vi "StateMachine.vi"() -> ()   [LabVIEW 2013, in "GP22_TDC_Arduinoed.lvlib"]
uses:
  GP22_TDC_Arduinoed.lvlib
  typedefs/State.ctl
  typedefs/Data.ctl
  <vilib>/Utility/file.llb/Write To Spreadsheet File (DBL).vi
  Public/Globals.vi
  <vilib>/Analysis/NI_AALBase.lvlib
panel:
  in  "VISA resource name":refnum<visa-resource-name>
  in  "Exit":bool
  in  "Tab Control":T1(tab)
  in  "Start calibration":bool
  in  "Save data":bool
  in  "Number of calibration readings":i32=100
  out "Histogram":dynamicdata(graph)
  out "Standard deviation":dbl format="%^_2g"
  out "Mean":dbl format="%^_4g"
  out "Calibration readings":dbl[](array[numeric])
  in  "Wait time (ms)":u32=10
  out "Progress":u8(slide) scale=0.0..100.0
  in  "Auto calibrate? (false)":bool
  in  "Double resolution? (false)":bool
  out "Freq / Hz":dbl format="%^#_6g"
  out "output / s":dbl format="%^#_6g"
  in  "Single Measurement":bool caption="Measure"
  out "MMProgress":u8(slide) scale=0.0..100.0
  out "output/s":dbl[](array[numeric]) format="%^#_6g"
  out "Raw output":dbl[](array[numeric])
  out "Calibration":dbl[](array[numeric])
  out "Multiple Meas. Histogram":dynamicdata(graph) caption="Histogram"
  in  "Time / ms (30000)":u32=30000
  out "Size":i32
  out "Mean Freq / Hz":dbl format="%^#_6g"
  out "Time frac. S.D.":dbl format="%^#_6e"
  out "Mean Time / s":dbl format="%^.3e"
  in  "Time between calibrations (ms)":u32=1000
  in  "Multiple Measurements":bool caption="Measure"
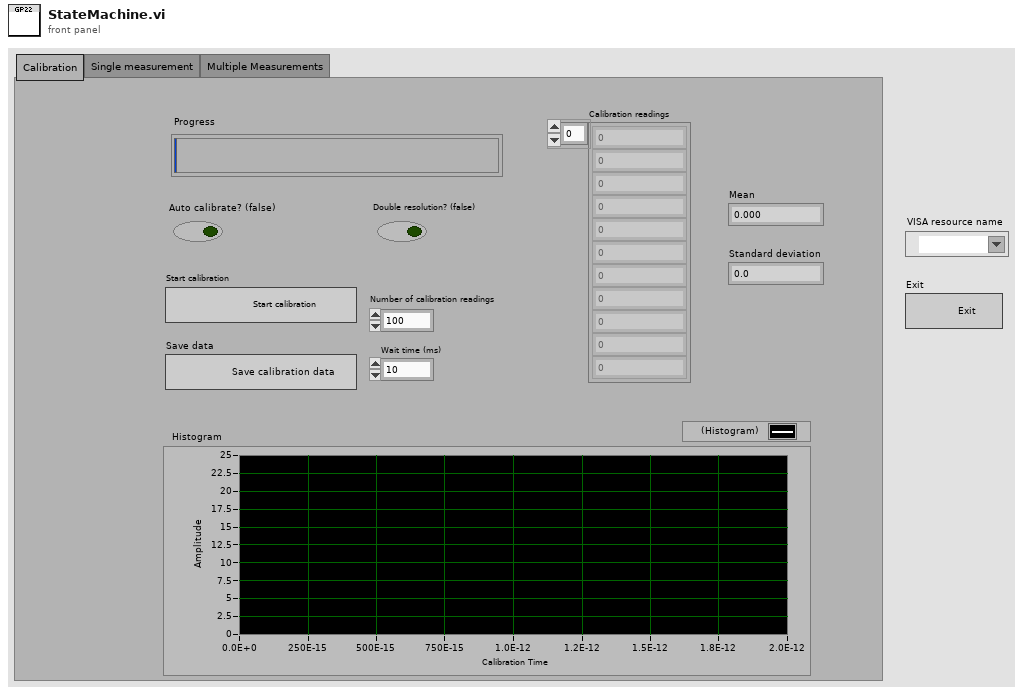
[diagram p1: front panel]
types:
  T1 = enum32{"Calibration", "Single measurement", "Multiple Measurements"}
  T2 = typedef "GP22_TDC_Arduinoed.lvlib/Data.ctl" = cluster{"VISA resource name":refnum<visa-resource-name>}
  T3 = typedef "GP22_TDC_Arduinoed.lvlib/State.ctl" = enum16{"Initialize", "Wait for Event", "Multiple Measurements", "Take calibration data", "Save calibration data", "Single measurement", "Exit"}
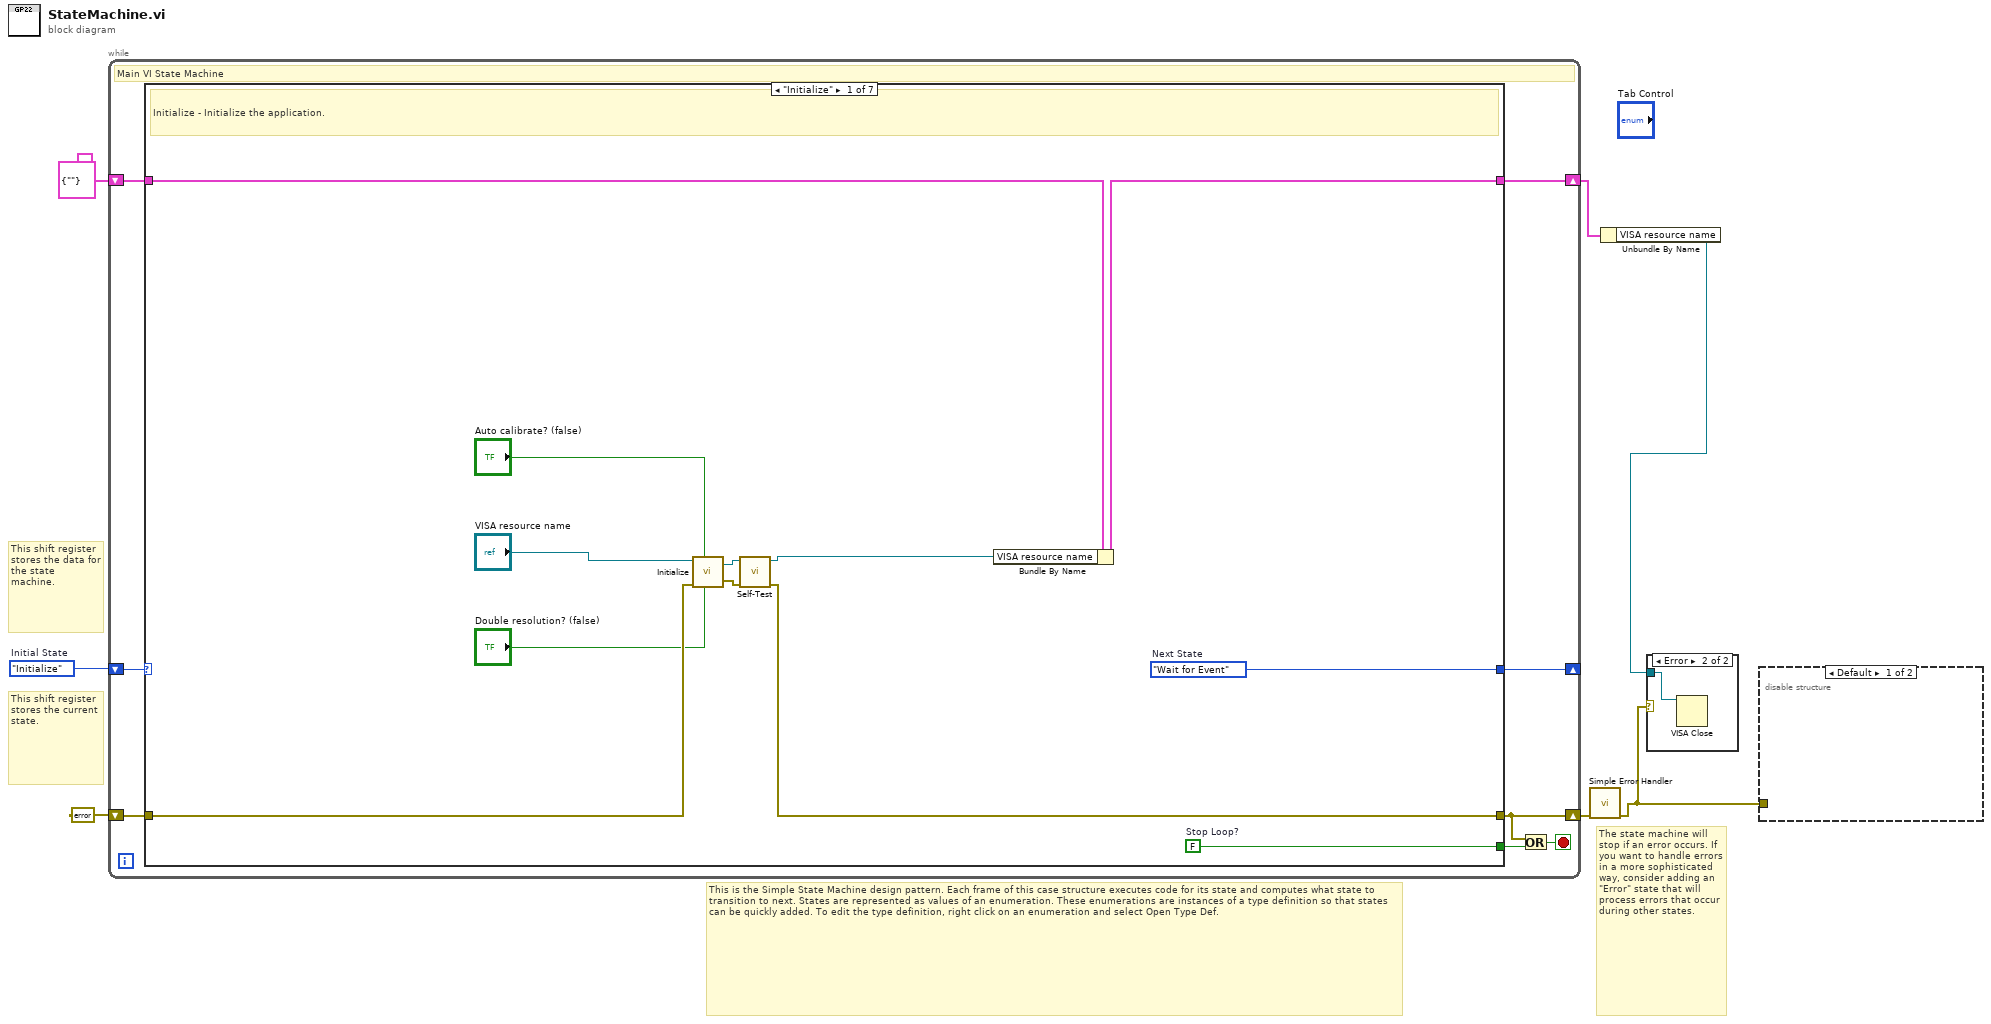
[diagram p0: block diagram]
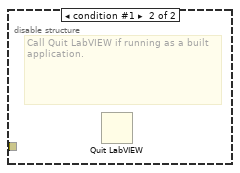
[diagram p3: hidden frame]
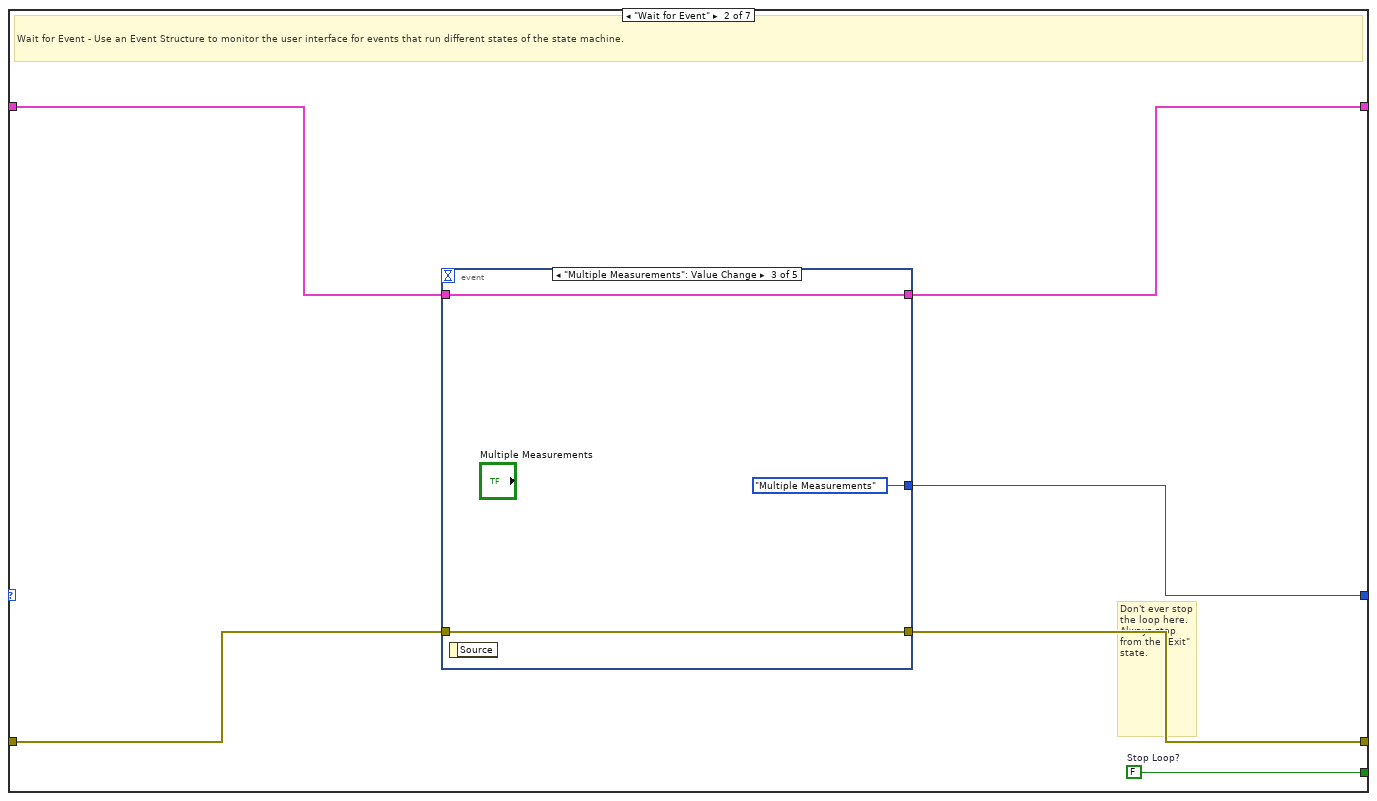
[diagram p4: hidden frame]
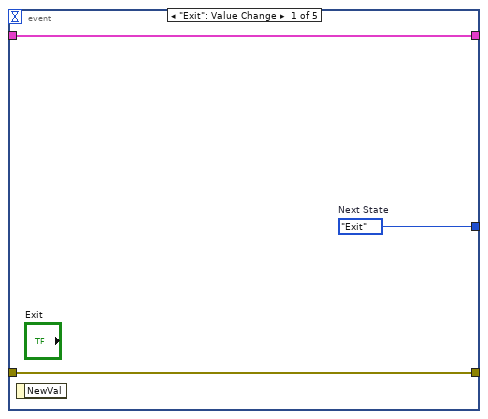
[diagram p5: hidden frame]
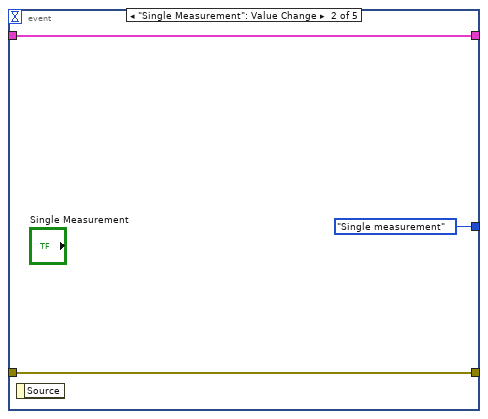
[diagram p6: hidden frame]
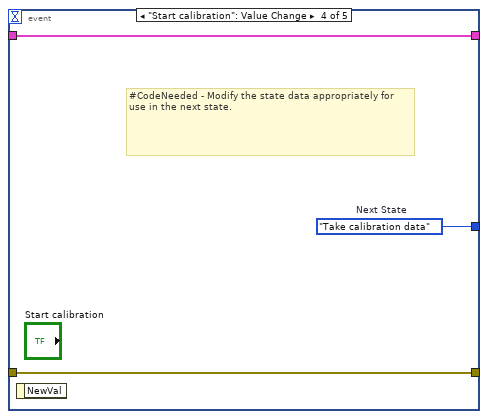
[diagram p7: hidden frame]
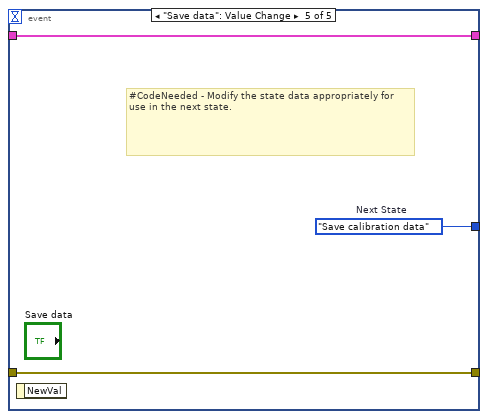
[diagram p8: hidden frame]
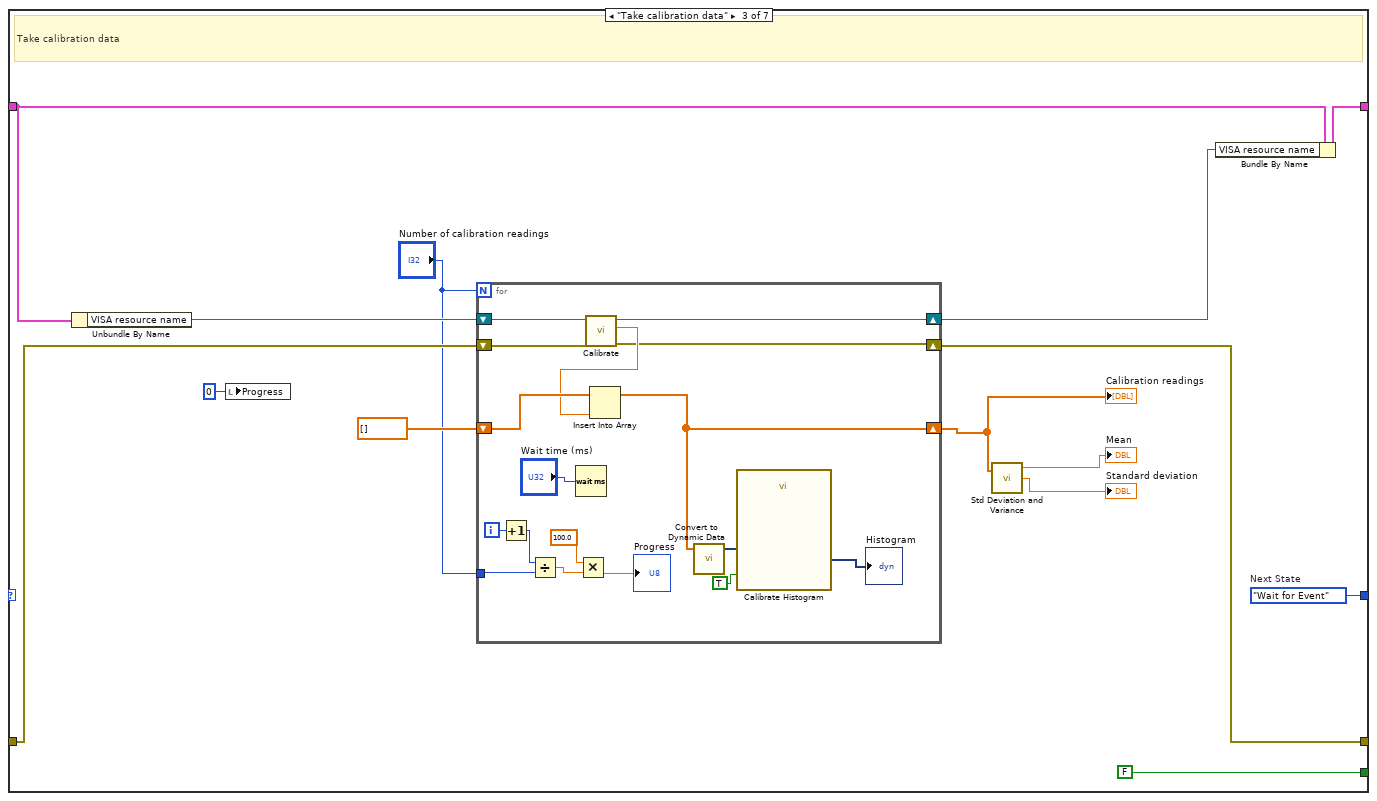
[diagram p9: hidden frame]
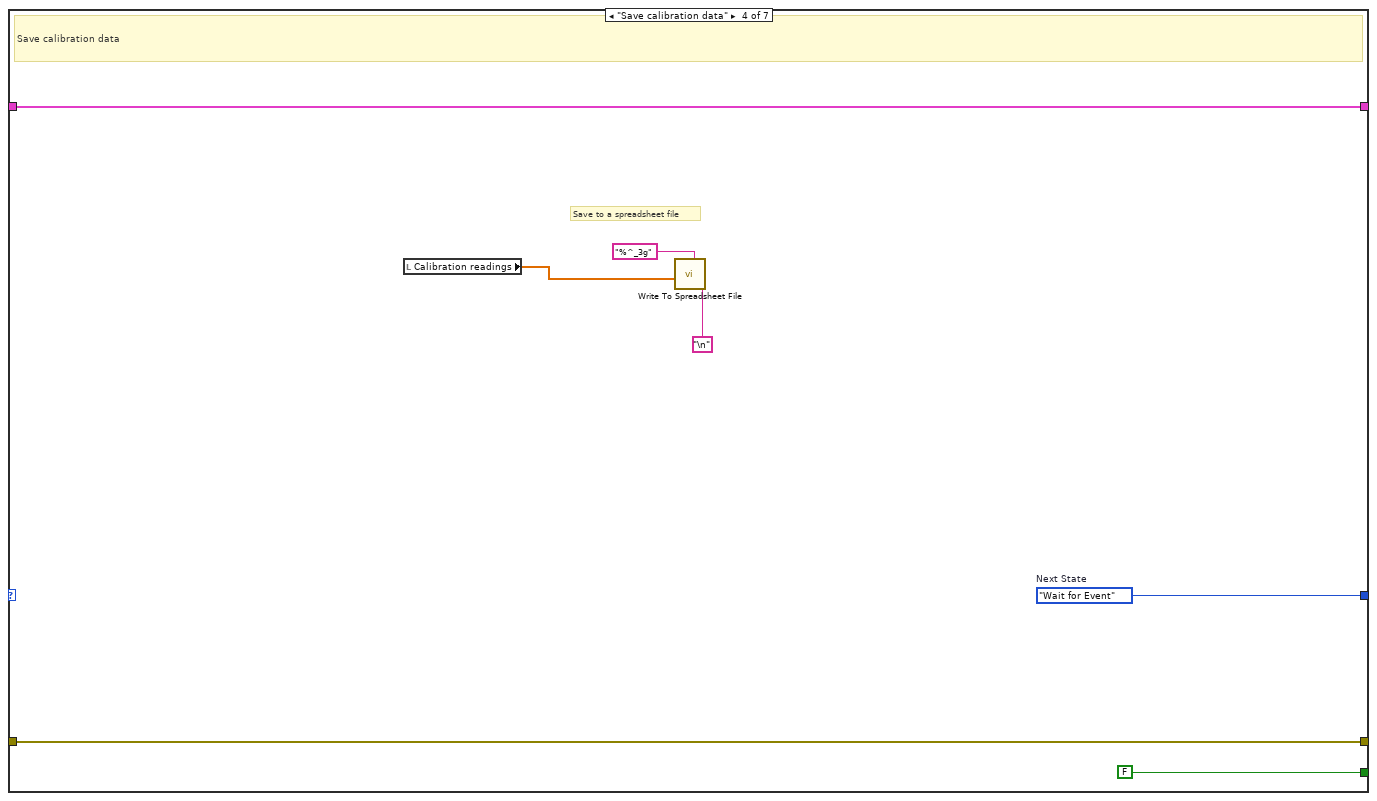
[diagram p10: hidden frame]
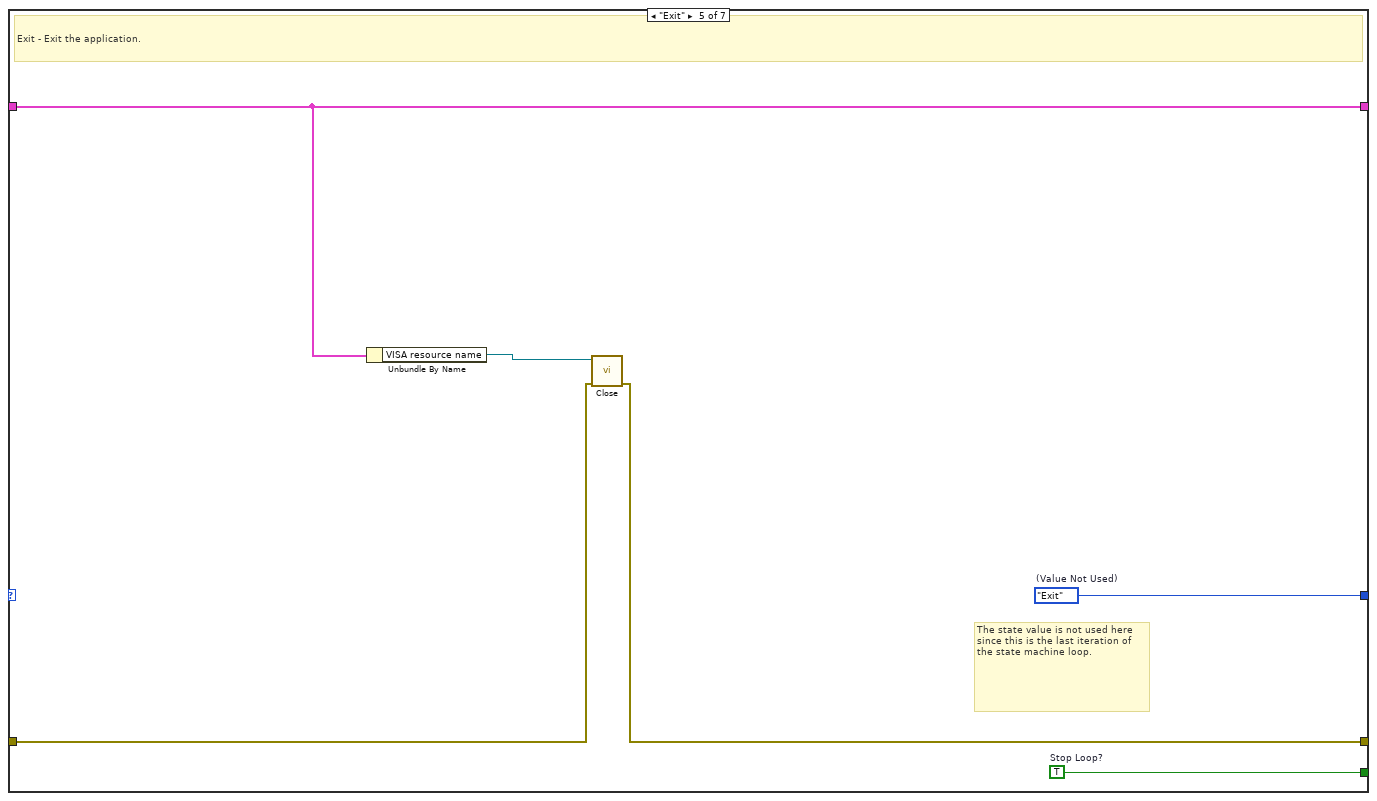
[diagram p11: hidden frame]
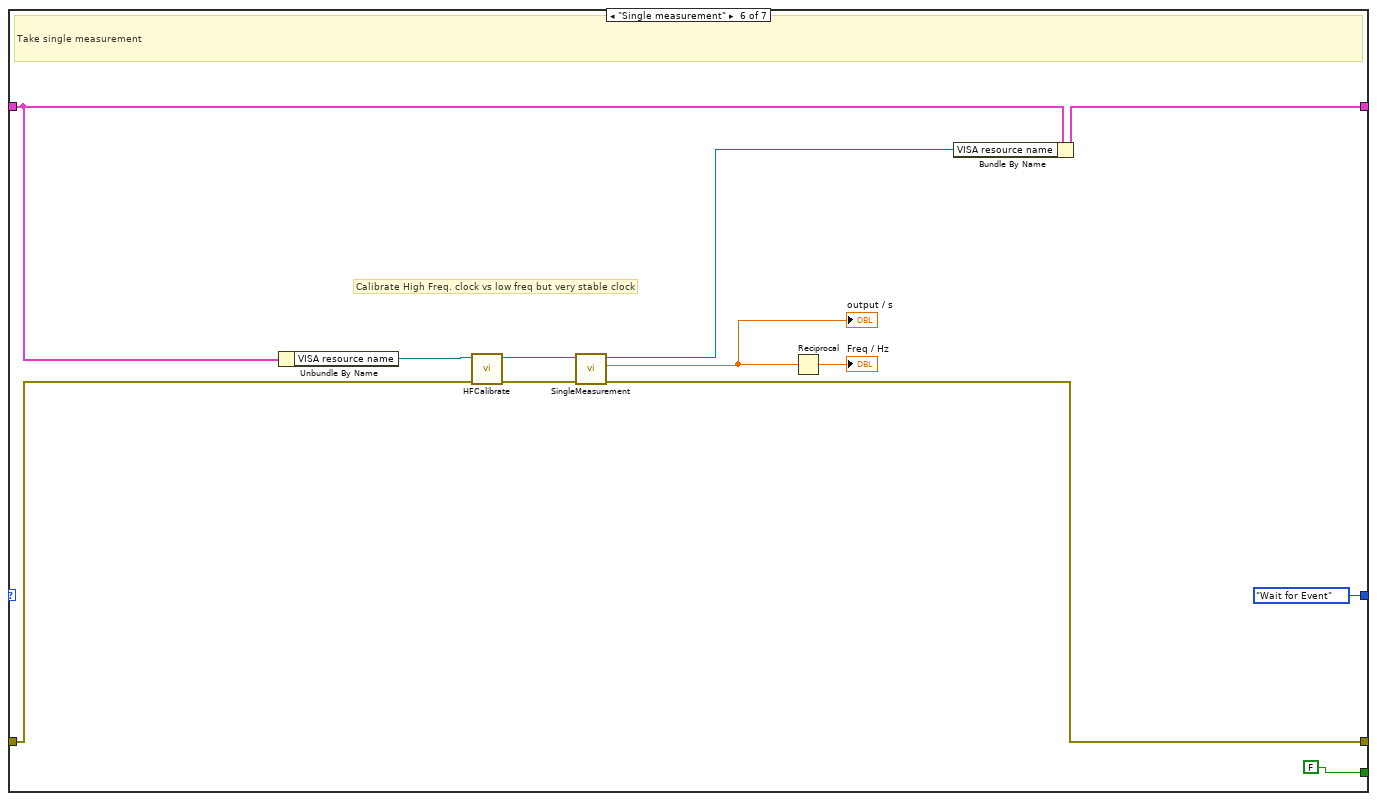
[diagram p12: hidden frame]
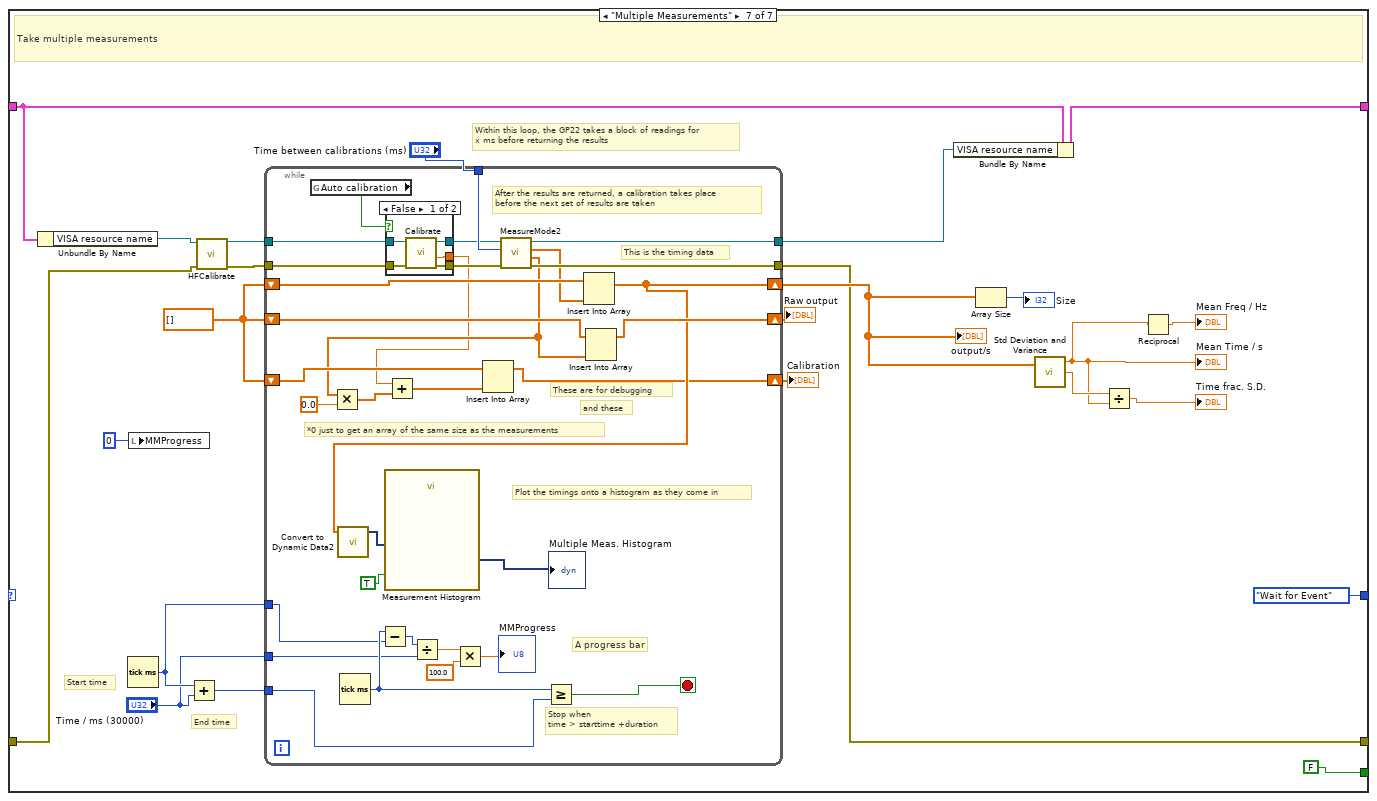
[diagram p13: hidden frame]
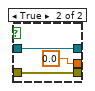
[diagram p14: hidden frame]
diagram:
  w7 = State."Initialize"  # Initial State
  # "The state machine will stop if an error occurs. If you want to handle errors in a more sophisticated way, consider adding an \"Error\" state that will process errors that occur during other states."
  # "This shift register stores the data for the state machine."
  # "This is the Simple State Machine design pattern. Each frame of this case structure executes code for its state and computes what state to transition to next. States are represented as values of an enumeration. These enumerations are instances of a type definition so that states can be quickly added. To edit the type definition, right click on an enumeration and select Open Type Def."
  # "This shift register stores the current state."
  n1 = while {
    shift-right: [w14] -> _
    shift-left: w7 -> [w15]
    shift-right: [w12] -> w3
    shift-left: T2 {"VISA resource name"=""} ("Data") -> [w13]
    shift-right: [w8] -> w4
    shift-left: errorcluster {"status"=FALSE, "code"=0, "source"=""} ("error constant") -> [w11]
    stop <- w9 stop-if-true
    # "Main VI State Machine"
    n2 = case shown="\"Initialize\"" w15 {
      tunnel: [w27 w33 w62 w86 w92 State."Wait for Event" ("(Value Not Used)") State."Wait for Event" ("(Value Not Used)")] -> w14
      tunnel: [w26 w32 FALSE ("Stop Loop?") FALSE ("Stop Loop?") w91 FALSE ("Stop Loop?") FALSE ("Stop Loop?")] -> w10
      tunnel: w13 -> [w25 w31 w59 w84 w90 w102 w128]
      tunnel: [w24 w30 w55 w84 w90 w101 w127] -> w12
      tunnel: w11 -> [w19 w29 w57 w83 w88 w93 w108]
      tunnel: [w18 w28 w56 w83 w87 w100 w112] -> w8
      frame "Initialize" {
        w26 = FALSE  # Stop Loop?
        w27 = State."Wait for Event"  # Next State
        # "Initialize - Initialize the application."
        n3 = call "Initialize.vi"("Double resolution? (false)"="Double resolution? (false)", "Auto calibrate? (false)"="Auto calibrate? (false)", "error in (no error)"=w19, "VISA resource name"="VISA resource name") -> ("error out"=w20:errorcluster, "VISA resource name out"=w22:refnum<visa-resource-name>)  [unwired: 2 in]
        n4 = call "Self-Test.vi"("error in (no error)"=w20, "VISA resource name"=w22) -> ("error out"=w18:errorcluster, "VISA resource name out"=w21:refnum<visa-resource-name>)  [unwired: 6 in, 2 out]
        n5 = Bundle By Name(cluster=w25, "VISA resource name"=w21) -> (w24:T2)
      }
      frame "Wait for Event" {
        w32 = FALSE  # Stop Loop?
        # "Don't ever stop the loop here. Always stop from the \"Exit\" state."
        # "Wait for Event - Use an Event Structure to monitor the user interface for events that run different states of the state machine."
        n6 = event shown="[2] \"Multiple Measurements\": Value Change" {
          selector: _ -> [_ _ _ _ _]
          dyn-events: _ -> [_ _ _ _ _]
          timeout: _ -> [_ _ _ _ _]
          tunnel: [w36 State."Single measurement" ("Next State") State."Multiple Measurements" ("Next State") w45 w48] -> w33
          tunnel: w31 -> [w35 w39 w42 w43 w46]
          tunnel: [w35 w39 w42 w43 w46] -> w30
          tunnel: w29 -> [w34 w38 w41 w44 w47]
          tunnel: [w34 w38 w41 w44 w47] -> w28
          event "Exit": Value Change {
            w36 = State."Exit"  # Next State
            n7 = event-data() -> ()  [unwired: 1 in, 1 out]
          }
          event "Single Measurement": Value Change {
            n8 = event-data() -> ()  [unwired: 1 in, 1 out]
          }
          event "Multiple Measurements": Value Change {
            n9 = event-data() -> ()  [unwired: 1 in, 1 out]
          }
          event "Start calibration": Value Change {
            w45 = State."Take calibration data"  # Next State
            # "#CodeNeeded - Modify the state data appropriately for use in the next state."
            n10 = event-data() -> ()  [unwired: 1 in, 1 out]
          }
          event "Save data": Value Change {
            w48 = State."Save calibration data"  # Next State
            # "#CodeNeeded - Modify the state data appropriately for use in the next state."
            n11 = event-data() -> ()  [unwired: 1 in, 1 out]
          }
        }
      }
      frame "Take calibration data" {
        w62 = State."Wait for Event"  # Next State
        # "Take calibration data"
        n12 = Unbundle By Name(w59) -> ("VISA resource name"=w58:refnum<visa-resource-name>)
        n13 = local write "Progress"(u8 0 ("Progress")) -> ()
        n14 = for {
          N: "Number of calibration readings" -> [_]
          shift-right: [w63] -> w50
          shift-left: dbl[] [] -> [w76]
          shift-right: [w73] -> w56
          shift-left: w57 -> [w78]
          shift-right: [w74] -> w54
          shift-left: w58 -> [w79]
          tunnel: "Number of calibration readings" -> [w70]
          i -> [w71]
          n15 = Increment(x=w71) -> (x+1=w67:i32)
          n16 = Divide(x=w67, y=w70) -> (x/y=w72:dbl)
          n17 = Wait (ms)(milliseconds to wait="Wait time (ms)") -> ()  [unwired: 1 out]
          n18 = Multiply(x=100.0, y=w72) -> (x*y=→"Progress":dbl)
          n19 = call "Calibrate.vi"("error in (no error)"=w78, "VISA resource name"=w79) -> ("error out"=w73:errorcluster, "output / s"=w75:dbl, "VISA resource name out"=w74:refnum<visa-resource-name>)  [unwired: 5 in, 1 out]
          n20 = Insert Into Array(array=w76, new element=w75) -> (w63:dbl[])  [unwired: 1 in]
          n21 = call "Convert to Dynamic Data"("Array"=w63) -> ("Dynamic Data Type"=w64:dynamicdata)  [unwired: 3 in]
          n22 = call "Calibrate Histogram"("Reset"=TRUE, "Signal"=w64) -> ("Histogram"=→"Histogram":dynamicdata)  [unwired: 8 in, 1 out]
        }
        "Calibration readings" <- w50
        n23 = call <vilib>:"Std Deviation and Variance.vi"("X"=w50) -> ("mean"=→"Mean":dbl, "standard deviation"=→"Standard deviation":dbl)  [unwired: 1 in, 1 out]
        n24 = Bundle By Name(cluster=w59, "VISA resource name"=w54) -> (w55:T2)
      }
      frame "Save calibration data" {
        w86 = State."Wait for Event"  # Next State
        # "Save to a spreadsheet file"
        # "Save calibration data"
        n25 = local read "Calibration readings"() -> (w82:dbl[])
        n26 = call-poly <vilib>:"Write To Spreadsheet File.vi"("delimiter (\\t)"="\n" ("delimiter (\\t)"), "format (%.3f)"="%^_3g", "1D data"=w82) -> ()  [unwired: 5 in, 1 out]
      }
      frame "Exit" {
        w91 = TRUE  # Stop Loop?
        w92 = State."Exit"  # (Value Not Used)
        # "The state value is not used here since this is the last iteration of the state machine loop."
        # "Exit - Exit the application."
        n27 = Unbundle By Name(w90) -> ("VISA resource name"=w89:refnum<visa-resource-name>)
        n28 = call "Close.vi"("error in (no error)"=w88, "VISA resource name"=w89) -> ("error out"=w87:errorcluster)  [unwired: 9 in]
      }
      frame "Single measurement" {
        # "Calibrate High Freq. clock vs low freq but very stable clock"
        # "Take single measurement"
        n29 = Unbundle By Name(w102) -> ("VISA resource name"=w96:refnum<visa-resource-name>)
        n30 = call "HFCalibrate.vi"("error in (no error)"=w93, "VISA resource name"=w96) -> ("error out"=w94:errorcluster, "VISA resource name out"=w95:refnum<visa-resource-name>)  [unwired: 5 in, 2 out]
        n31 = call "SingleMeasurement.vi"("error in (no error)"=w94, "VISA resource name"=w95) -> ("error out"=w100:errorcluster, "output / s"=w103:dbl, "VISA resource name out"=w99:refnum<visa-resource-name>)  [unwired: 7 in]
        "output / s" <- w103
        n32 = Reciprocal(x=w103) -> (1/x=→"Freq / Hz":dbl)
        n33 = Bundle By Name(cluster=w102, "VISA resource name"=w99) -> (w101:T2)
      }
      frame "Multiple Measurements" {
        w115 = dbl[] [] ("output")
        # "Within this loop, the GP22 takes a block of readings for\nx ms before returning the results"
        # "End time"
        # "Start time"
        # "Take multiple measurements"
        n34 = Unbundle By Name(w128) -> ("VISA resource name"=w109:refnum<visa-resource-name>)
        n35 = Tick Count (ms)() -> (millisecond timer value=w106:u32)
        n36 = local write "MMProgress"(u8 0 ("MMProgress")) -> ()
        n37 = Add(x=w106, y="Time / ms (30000)") -> (x+y=w118:u32)
        n38 = call "HFCalibrate.vi"("error in (no error)"=w108, "VISA resource name"=w109) -> ("error out"=w110:errorcluster, "VISA resource name out"=w111:refnum<visa-resource-name>)  [unwired: 5 in, 2 out]
        n39 = while {
          tunnel: w111 -> [w156]
          tunnel: [w160] -> w113
          tunnel: "Time between calibrations (ms)" -> [w159]
          tunnel: w110 -> [w155]
          tunnel: [w158] -> w112
          tunnel: w118 -> [w141]
          shift-right: [w138] -> w122
          shift-left: w115 -> [w152]
          shift-right: [w148] -> w116
          shift-left: w115 -> [w149]
          shift-right: [w129] -> w114
          shift-left: w115 -> [w147]
          tunnel: w106 -> [w135]
          tunnel: "Time / ms (30000)" -> [w133]
          stop <- w157 stop-if-true
          # "A progress bar"
          # "Plot the timings onto a histogram as they come in"
          # "and these"
          # "These are for debugging"
          # "This is the timing data"
          # "After the results are returned, a calibration takes place\nbefore the next set of results are taken"
          # "*0 just to get an array of the same size as the measurements"
          # "Stop when \ntime > starttime +duration"
          n40 = global read "Globals.vi" "Auto calibration"() -> (w150:bool)
          n41 = Tick Count (ms)() -> (millisecond timer value=w136:u32)
          n42 = Subtract(x=w136, y=w135) -> (x-y=w134:u32)
          n43 = case shown="False" w150 {
            tunnel: w156 -> [w165 w168]
            tunnel: w155 -> [w164 w167]
            tunnel: [w163 w167] -> w154
            tunnel: [w162 w168] -> w153
            tunnel: [w161 0.0 ("y")] -> w143
            frame False {
              n44 = call "Calibrate.vi"("error in (no error)"=w164, "VISA resource name"=w165) -> ("error out"=w163:errorcluster, "output raw"=w161:dbl, "VISA resource name out"=w162:refnum<visa-resource-name>)  [unwired: 5 in, 1 out]
            }
            frame True {
            }
          }
          n45 = Divide(x=w134, y=w133) -> (x/y=w132:dbl)
          n46 = Multiply(x=w132, y=100.0) -> (x*y=→"MMProgress":dbl)
          n47 = call "MeasureMode2.vi"("error in (no error)"=w154, "Time in ms (30000)"=w159, "VISA resource name"=w153) -> ("error out"=w158:errorcluster, "Raw output"=w146:dbl[], "output/s"=w151:dbl[], "VISA resource name out"=w160:refnum<visa-resource-name>)  [unwired: 5 in]
          n48 = Multiply(x=w146, y=0.0) -> (x*y=w144:dbl[])
          n49 = Add(x=w143, y=w144) -> (x+y=w142:dbl[])
          n50 = Insert Into Array(array=w147, new element=w142) -> (w129:dbl[])  [unwired: 1 in]
          n51 = Greater Or Equal?(x=w136, y=w141) -> (x >= y?=w157:bool)
          n52 = Insert Into Array(array=w152, new element=w151) -> (w138:dbl[])  [unwired: 1 in]
          n53 = call "Convert to Dynamic Data2"("Array"=w138) -> ("Dynamic Data Type"=w139:dynamicdata)  [unwired: 3 in]
          n54 = call "Measurement Histogram"("Reset"=TRUE, "Signal"=w139) -> ("Histogram"=→"Multiple Meas. Histogram":dynamicdata)  [unwired: 8 in, 1 out]
          n55 = Insert Into Array(array=w149, new element=w146) -> (w148:dbl[])  [unwired: 1 in]
        }
        "output/s" <- w122
        "Raw output" <- w116
        "Calibration" <- w114
        n56 = Bundle By Name(cluster=w128, "VISA resource name"=w113) -> (w127:T2)
        n57 = Array Size(array=w122) -> (size(s)=→"Size":i32)
        n58 = call <vilib>:"Std Deviation and Variance.vi"("X"=w122) -> ("mean"=w119:dbl, "standard deviation"=w121:dbl)  [unwired: 1 in, 1 out]
        "Mean Time / s" <- w119
        n59 = Divide(x=w121, y=w119) -> (x/y=→"Time frac. S.D.":dbl)
        n60 = Reciprocal(x=w119) -> (1/x=→"Mean Freq / Hz":dbl)
      }
    }
    n61 = Or(x=w8, y=w10) -> (x .or. y?=w9:bool)
  }
  n62 = call <vilib>:"Simple Error Handler.vi"("error in (no error)"=w4) -> ("error out"=w1:errorcluster)  [unwired: 4 in, 4 out]
  n63 = Unbundle By Name(w3) -> ("VISA resource name"=w2:refnum<visa-resource-name>)
  n64 = case shown="Error" w1 {
    tunnel: w2 -> [_ w169]
    frame No Error {
    }
    frame Error {
      n65 = VISA Close(VISA resource name=w169) -> ()  [unwired: 1 in, 1 out]
    }
  }
  n66 = disable-structure shown="Default" {
    disable-tunnel: w1 -> [_ _]
    frame condition #0 (active) {
    }
    frame condition #1 {
      # "Call Quit LabVIEW if running as a built application."
      n67 = Quit LabVIEW() -> ()  [unwired: 1 in]
    }
  }
